vi "Validate Sink Settings.vi"(8 "error in (no error)":errorcluster, 11 "Text File Sink in":refnum<class "Text File Sink.lvclass">) -> (0 "error out":errorcluster, 3 "Text File Sink out":refnum<class "Text File Sink.lvclass">)   [LabVIEW 2018, in "MVA Framework.lvlib" / "Text File Sink.lvclass"]
uses:
  Text File Sink.lvclass
  <vilib>/ErrorRing/Error Ring.xnode
  <vilib>/Utility/error.llb/Error Cluster From Error Code.vi
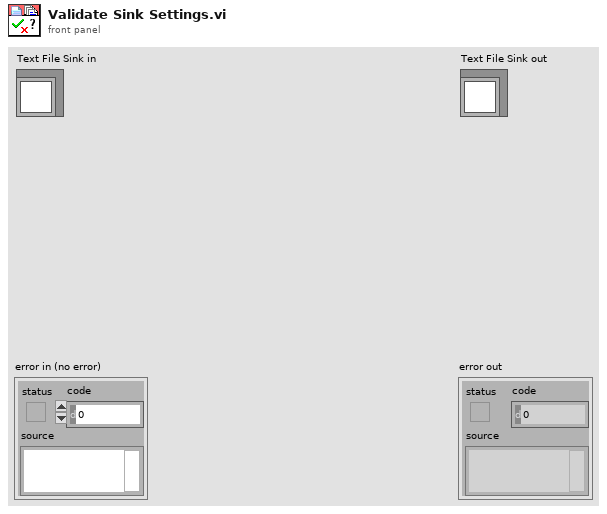
[diagram p1: front panel]
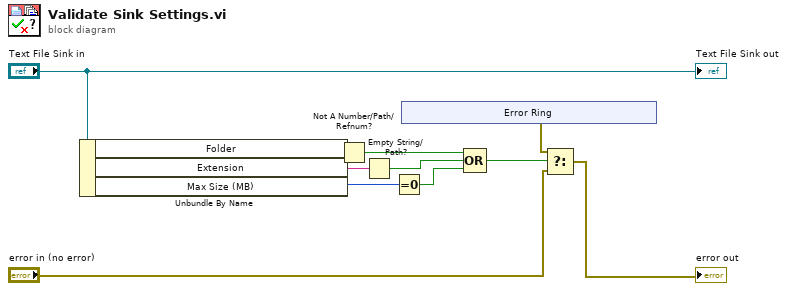
[diagram p0: block diagram]
diagram:
  n1 = Unbundle By Name("Text File Sink in") -> ("Folder"=w10:path, "Extension"=w9:string, "Max Size (MB)"=w8:i64)
  n2 = Not A Number/Path/Refnum?(number/path/refnum=w10) -> (NaN/Path/Refnum?=w7:bool)
  n3 = Empty String/Path?(string/path=w9) -> (empty?=w6:bool)
  n4 = Equal To 0?(x=w8) -> (x = 0?=w5:bool)
  n5 = xnode "Error Ring"() -> ("错误输出"=w1:errorcluster)
  n6 = Compound Arithmetic op=OR(w7, w6, w5) -> (w4:bool)
  n7 = Select(t=w1, s=w4, f="error in (no error)") -> (s? t:f=→"error out":errorcluster)
  "Text File Sink out" <- "Text File Sink in"
